vi "cRIO Vendor and Components Library.vi"() -> (0 "List of Modules":T4[](array[typedef])=[{"Module ID"=0, "Module Name"=""}, {"Module ID"=28836, "Module Name"="NI 9201"}, {"Module ID"=29089, "Module Name"="NI 9201 DSUB"}, {"Module ID"=29851, "Module Name"="NI 9201E"}, {"Module ID"=29853, "Module Name"="NI 9201E DSUB"}, {"Module ID"=28969, "Module Name"="NI 9203"}, {"Module ID"=29707, "Module Name"="NI 9203E"}, {"Module ID"=29162, "Module Name"="NI 9205"}, {"Module ID"=28970, "Module Name"="NI 9205 DSUB"}, {"Module ID"=29771, "Module Name"="NI 9205E"}, {"Module ID"=29163, "Module Name"="NI 9206"}, {"Module ID"=28835, "Module Name"="NI 9211"}, {"Module ID"=29706, "Module Name"="NI 9211E"}, {"Module ID"=29769, "Module Name"="NI 9213"}, {"Module ID"=29754, "Module Name"="NI 9213E"}, {"Module ID"=29934, "Module Name"="NI 9214"}, {"Module ID"=28838, "Module Name"="NI 9215"}, {"Module ID"=28981, "Module Name"="NI 9215 BNC"}, {"Module ID"=29709, "Module Name"="NI 9215E"}, {"Module ID"=29789, "Module Name"="NI 9215E BNC"}, {"Module ID"=28971, "Module Name"="NI 9217"}, {"Module ID"=29452, "Module Name"="NI 9219"}, {"Module ID"=29551, "Module Name"="NI 9219 LEMO"}, {"Module ID"=29761, "Module Name"="NI 9219E"}, {"Module ID"=29664, "Module Name"="NI 9220"}, {"Module ID"=30229, "Module Name"="NI 9220 DSUB"}, {"Module ID"=29841, "Module Name"="NI 9220E"}, {"Module ID"=28837, "Module Name"="NI 9221"}, {"Module ID"=29090, "Module Name"="NI 9221 DSUB"}, {"Module ID"=29852, "Module Name"="NI 9221E"}, {"Module ID"=29854, "Module Name"="NI 9221E DSUB"}, {"Module ID"=29571, "Module Name"="NI 9225"}, {"Module ID"=29704, "Module Name"="NI 9225E"}, {"Module ID"=29718, "Module Name"="NI 9227"}, {"Module ID"=29772, "Module Name"="NI 9227E"}, {"Module ID"=29437, "Module Name"="NI 9229"}, {"Module ID"=29544, "Module Name"="NI 9229 BNC"}, {"Module ID"=29725, "Module Name"="NI 9229E"}, {"Module ID"=28840, "Module Name"="NI 9233"}, {"Module ID"=29365, "Module Name"="NI 9234"}, {"Module ID"=29882, "Module Name"="NI 9234"}, {"Module ID"=30042, "Module Name"="NI 9234E"}, {"Module ID"=29482, "Module Name"="NI 9235"}, {"Module ID"=29898, "Module Name"="NI 9235E"}, {"Module ID"=29483, "Module Name"="NI 9236"}, {"Module ID"=29899, "Module Name"="NI 9236E"}, {"Module ID"=29123, "Module Name"="NI 9237"}, {"Module ID"=29604, "Module Name"="NI 9237 DSUB"}, {"Module ID"=29727, "Module Name"="NI 9237E"}, {"Module ID"=29774, "Module Name"="NI 9237E DSUB"}, {"Module ID"=29122, "Module Name"="NI 9239"}, {"Module ID"=29543, "Module Name"="NI 9239 BNC"}, {"Module ID"=29724, "Module Name"="NI 9239E"}, {"Module ID"=28839, "Module Name"="NI 9263"}, {"Module ID"=29545, "Module Name"="NI 9263 BNC"}, {"Module ID"=29726, "Module Name"="NI 9263E"}, {"Module ID"=29430, "Module Name"="NI 9264"}, {"Module ID"=29788, "Module Name"="NI 9264 DSUB"}, {"Module ID"=29767, "Module Name"="NI 9264E"}, {"Module ID"=29787, "Module Name"="NI 9264E DSUB"}, {"Module ID"=28972, "Module Name"="NI 9265"}, {"Module ID"=29762, "Module Name"="NI 9265E"}, {"Module ID"=29444, "Module Name"="NI 9375"}, {"Module ID"=29818, "Module Name"="NI 9375 DSUB"}, {"Module ID"=29802, "Module Name"="NI 9375E"}, {"Module ID"=29819, "Module Name"="NI 9375E DSUB"}, {"Module ID"=30274, "Module Name"="NI 9381"}, {"Module ID"=30272, "Module Name"="NI 9381 DSUB"}, {"Module ID"=28976, "Module Name"="NI 9401"}, {"Module ID"=29480, "Module Name"="NI 9402"}, {"Module ID"=28977, "Module Name"="NI 9403"}, {"Module ID"=29708, "Module Name"="NI 9403E"}, {"Module ID"=28829, "Module Name"="NI 9411"}, {"Module ID"=28831, "Module Name"="NI 9421"}, {"Module ID"=28974, "Module Name"="NI 9421 DSUB"}, {"Module ID"=29130, "Module Name"="NI 9422"}, {"Module ID"=28830, "Module Name"="NI 9423"}, {"Module ID"=28975, "Module Name"="NI 9425"}, {"Module ID"=29546, "Module Name"="NI 9426"}, {"Module ID"=30017, "Module Name"="NI 9426E"}, {"Module ID"=28828, "Module Name"="NI 9435"}, {"Module ID"=30128, "Module Name"="NI 9467"}, {"Module ID"=29907, "Module Name"="NI 9469"}, {"Module ID"=28833, "Module Name"="NI 9472"}, {"Module ID"=28978, "Module Name"="NI 9472 DSUB"}, {"Module ID"=28832, "Module Name"="NI 9474"}, {"Module ID"=29559, "Module Name"="NI 9475"}, {"Module ID"=28979, "Module Name"="NI 9476"}, {"Module ID"=29131, "Module Name"="NI 9477"}, {"Module ID"=29466, "Module Name"="NI 9478"}, {"Module ID"=29755, "Module Name"="NI 9478E"}, {"Module ID"=28834, "Module Name"="NI 9481"}, {"Module ID"=29705, "Module Name"="NI 9481E"}, {"Module ID"=29174, "Module Name"="NI 9485"}, {"Module ID"=29165, "Module Name"="NI 9505"}, {"Module ID"=29857, "Module Name"="NI 9505E"}, {"Module ID"=29645, "Module Name"="NI 9512"}, {"Module ID"=29646, "Module Name"="NI 9514"}, {"Module ID"=29648, "Module Name"="NI 9516"}, {"Module ID"=28980, "Module Name"="NI 9802"}, {"Module ID"=29171, "Module Name"="NI 9852"}, {"Module ID"=29007, "Module Name"="NI 9853"}, {"Module ID"=29820, "Module Name"="NI 9861"}, {"Module ID"=29821, "Module Name"="NI 9862"}, {"Module ID"=29824, "Module Name"="NI 9866"}, {"Module ID"=29445, "Module Name"="NI 9870"}, {"Module ID"=29759, "Module Name"="NI 9870E"}, {"Module ID"=29446, "Module Name"="NI 9871"}, {"Module ID"=29760, "Module Name"="NI 9871E"}, {"Module ID"=29826, "Module Name"="NI 9881"}, {"Module ID"=29827, "Module Name"="NI 9882"}, {"Module ID"=29850, "Module Name"="NI 9882"}, {"Module ID"=29765, "Module Name"="NI 9222"}, {"Module ID"=30515, "Module Name"="NI 9222 BNC"}, {"Module ID"=29766, "Module Name"="NI 9222E"}, {"Module ID"=29932, "Module Name"="NI 9223"}, {"Module ID"=30516, "Module Name"="NI 9223 BNC"}, {"Module ID"=29933, "Module Name"="NI 9223E"}, {"Module ID"=29729, "Module Name"="NI 9208"}, {"Module ID"=29868, "Module Name"="NI 9208 DSUB"}, {"Module ID"=29764, "Module Name"="NI 9208E"}, {"Module ID"=29867, "Module Name"="NI 9208E DSUB"}, {"Module ID"=29730, "Module Name"="NI 9207"}, {"Module ID"=29869, "Module Name"="NI 9207 DSUB"}, {"Module ID"=29866, "Module Name"="NI 9207E DSUB"}, {"Module ID"=29934, "Module Name"="NI 9214"}, {"Module ID"=30015, "Module Name"="NI 9232"}, {"Module ID"=30016, "Module Name"="NI 9232E"}, {"Module ID"=29717, "Module Name"="NI 9269"}, {"Module ID"=29773, "Module Name"="NI 9269E"}, {"Module ID"=29981, "Module Name"="NI 9501"}, {"Module ID"=29988, "Module Name"="NI 9501E"}, {"Module ID"=29982, "Module Name"="NI 9502"}, {"Module ID"=29989, "Module Name"="NI 9502E"}, {"Module ID"=30155, "Module Name"="NI 9795"}] {"Module ID" format="%.0x"}, 1 "List of Backplanes":T3(array[cluster])=[{"Backplane ID"=30549, "Backplane Name"=enum."cRIO-9030"}, {"Backplane ID"=30539, "Backplane Name"=enum."cRIO-9031"}, {"Backplane ID"=30517, "Backplane Name"=enum."cRIO-9033"}, {"Backplane ID"=30541, "Backplane Name"=enum."cRIO-9034"}, {"Backplane ID"=30683, "Backplane Name"=enum."cRIO-9035"}, {"Backplane ID"=30684, "Backplane Name"=enum."cRIO-9036"}, {"Backplane ID"=30649, "Backplane Name"=enum."cRIO-9038"}, {"Backplane ID"=30685, "Backplane Name"=enum."cRIO-9039"}, {"Backplane ID"=30528, "Backplane Name"=enum."cRIO-9063"}, {"Backplane ID"=30529, "Backplane Name"=enum."cRIO-9064"}, {"Backplane ID"=30530, "Backplane Name"=enum."cRIO-9065"}, {"Backplane ID"=30531, "Backplane Name"=enum."cRIO-9066"}, {"Backplane ID"=30532, "Backplane Name"=enum."cRIO-9067"}, {"Backplane ID"=30456, "Backplane Name"=enum."cRIO-9068"}, {"Backplane ID"=29127, "Backplane Name"=enum."cRIO-9072"}, {"Backplane ID"=29677, "Backplane Name"=enum."cRIO-9073"}, {"Backplane ID"=29341, "Backplane Name"=enum."cRIO-9074"}, {"Backplane ID"=30067, "Backplane Name"=enum."cRIO-9075"}, {"Backplane ID"=29991, "Backplane Name"=enum."cRIO-9076"}, {"Backplane ID"=29979, "Backplane Name"=enum."cRIO-9081"}, {"Backplane ID"=29980, "Backplane Name"=enum."cRIO-9082"}, {"Backplane ID"=28918, "Backplane Name"=enum."cRIO-9101"}, {"Backplane ID"=28766, "Backplane Name"=enum."cRIO-9102"}, {"Backplane ID"=28919, "Backplane Name"=enum."cRIO-9103"}, {"Backplane ID"=28920, "Backplane Name"=enum."cRIO-9104"}, {"Backplane ID"=29686, "Backplane Name"=enum."cRIO-9111"}, {"Backplane ID"=29687, "Backplane Name"=enum."cRIO-9112"}, {"Backplane ID"=29688, "Backplane Name"=enum."cRIO-9113"}, {"Backplane ID"=29689, "Backplane Name"=enum."cRIO-9114"}, {"Backplane ID"=29690, "Backplane Name"=enum."cRIO-9116"}, {"Backplane ID"=29691, "Backplane Name"=enum."cRIO-9118"}, {"Backplane ID"=30152, "Backplane Name"=enum."NI 9146"}, {"Backplane ID"=30540, "Backplane Name"=enum."NI 9147"}, {"Backplane ID"=29928, "Backplane Name"=enum."NI 9148"}, {"Backplane ID"=30542, "Backplane Name"=enum."NI 9149"}, {"Backplane ID"=30246, "Backplane Name"=enum."NI 9154"}, {"Backplane ID"=30247, "Backplane Name"=enum."NI 9155"}, {"Backplane ID"=30009, "Backplane Name"=enum."NI 9157"}, {"Backplane ID"=30010, "Backplane Name"=enum."NI 9159"}, {"Backplane ID"=29555, "Backplane Name"=enum."sbRIO-9601"}, {"Backplane ID"=29557, "Backplane Name"=enum."sbRIO-9602"}, {"Backplane ID"=30091, "Backplane Name"=enum."sbRIO-9605"}, {"Backplane ID"=30093, "Backplane Name"=enum."sbRIO-9606"}, {"Backplane ID"=29591, "Backplane Name"=enum."sbRIO-9611"}, {"Backplane ID"=29592, "Backplane Name"=enum."sbRIO-9612"}, {"Backplane ID"=30398, "Backplane Name"=enum."sbRIO-9623"}, {"Backplane ID"=30143, "Backplane Name"=enum."sbRIO-9626"}, {"Backplane ID"=29593, "Backplane Name"=enum."sbRIO-9631"}, {"Backplane ID"=29594, "Backplane Name"=enum."sbRIO-9632"}, {"Backplane ID"=30149, "Backplane Name"=enum."sbRIO-9633"}, {"Backplane ID"=30146, "Backplane Name"=enum."sbRIO-9636"}, {"Backplane ID"=29560, "Backplane Name"=enum."sbRIO-9641"}, {"Backplane ID"=29595, "Backplane Name"=enum."sbRIO-9642"}] {"Backplane ID" format="%.0x"}, 2 "List of Controllers":T1(array[cluster])=[{"Controller ID"=28767, "Controller Name"="cRIO-9002/9004"}, {"Controller ID"=29071, "Controller Name"="cRIO-9012"}, {"Controller ID"=29465, "Controller Name"="cRIO-9014"}, {"Controller ID"=29650, "Controller Name"="cRIO-9022/3"}, {"Controller ID"=29785, "Controller Name"="cRIO-9024/5"}, {"Controller ID"=30549, "Controller Name"="cRIO-9030"}, {"Controller ID"=30539, "Controller Name"="cRIO-9031"}, {"Controller ID"=30517, "Controller Name"="cRIO-9033"}, {"Controller ID"=30541, "Controller Name"="cRIO-9034"}, {"Controller ID"=30683, "Controller Name"="cRIO-9035"}, {"Controller ID"=30684, "Controller Name"="cRIO-9036"}, {"Controller ID"=30649, "Controller Name"="cRIO-9038"}, {"Controller ID"=30685, "Controller Name"="cRIO-9039"}, {"Controller ID"=30528, "Controller Name"="cRIO-9063"}, {"Controller ID"=30529, "Controller Name"="cRIO-9064"}, {"Controller ID"=30530, "Controller Name"="cRIO-9065"}, {"Controller ID"=30531, "Controller Name"="cRIO-9066"}, {"Controller ID"=30532, "Controller Name"="cRIO-9067"}, {"Controller ID"=30422, "Controller Name"="cRIO-9068"}, {"Controller ID"=29127, "Controller Name"="cRIO-9072"}, {"Controller ID"=29677, "Controller Name"="cRIO-9073"}, {"Controller ID"=29341, "Controller Name"="cRIO-9074"}, {"Controller ID"=29991, "Controller Name"="cRIO-9075/6"}, {"Controller ID"=30013, "Controller Name"="cRIO-9081/2"}, {"Controller ID"=29555, "Controller Name"="sbRIO-9601"}, {"Controller ID"=29557, "Controller Name"="sbRIO-9602"}, {"Controller ID"=30091, "Controller Name"="sbRIO-9605/6"}, {"Controller ID"=29591, "Controller Name"="sbRIO-9611"}, {"Controller ID"=29592, "Controller Name"="sbRIO-9612"}, {"Controller ID"=30142, "Controller Name"="sbRIO-9623"}, {"Controller ID"=30145, "Controller Name"="sbRIO-9626"}, {"Controller ID"=29593, "Controller Name"="sbRIO-9631"}, {"Controller ID"=29594, "Controller Name"="sbRIO-9632"}, {"Controller ID"=30149, "Controller Name"="sbRIO-9633"}, {"Controller ID"=30146, "Controller Name"="sbRIO-9636"}, {"Controller ID"=29560, "Controller Name"="sbRIO-9641"}, {"Controller ID"=29595, "Controller Name"="sbRIO-9642"}] {"Controller ID" format="%.0x"}, 3 "List of Vendors":cluster{"Vendor ID":u16, "Vendor Name":string}[](array[cluster])=[{"Vendor ID"=0, "Vendor Name"=""}, {"Vendor ID"=4243, "Vendor Name"="National Instruments"}, {"Vendor ID"=44884, "Vendor Name"="AFT Atlas Fahrzeugtechnik"}, {"Vendor ID"=18193, "Vendor Name"="S.E.A. Datentechnik"}, {"Vendor ID"=56852, "Vendor Name"="Drivven"}, {"Vendor ID"=21226, "Vendor Name"="Bluetechnix"}, {"Vendor ID"=59499, "Vendor Name"="SET"}, {"Vendor ID"=8211, "Vendor Name"="COMSOFT"}, {"Vendor ID"=12507, "Vendor Name"="Averna"}] {"Vendor ID" format="%.0x"})   [LabVIEW 2016]
uses:
  Module/Controls/ModuleInformation.ctl
  Module/Module.lvclass
  Chassis/Controls/ChassisInformation.ctl
  Chassis/Chassis.lvclass
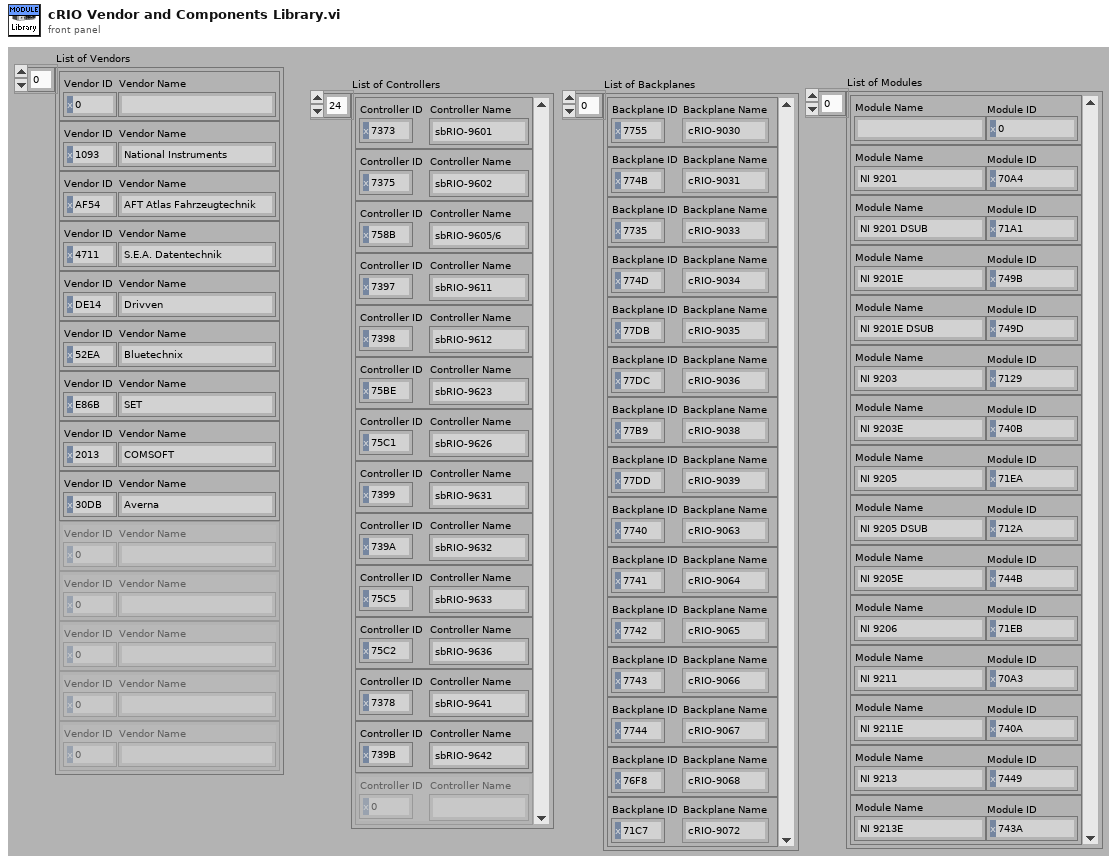
[diagram p1: front panel]
types:
  T1 = cluster{"Controller ID":u16, "Controller Name":string}[]
  T2 = typedef "cRIO Backplanes.ctl" = enum16{"<Undefined>", "cRIO-9030", "cRIO-9031", "cRIO-9033", "cRIO-9034", "cRIO-9035", "cRIO-9036", "cRIO-9038", "cRIO-9039", "cRIO-9063", "cRIO-9064", "cRIO-9065", "cRIO-9066", "cRIO-9067", "cRIO-9068", "cRIO-9072", "cRIO-9073", "cRIO-9074", "cRIO-9075", "cRIO-9076", "cRIO-9081", "cRIO-9082", "cRIO-9101", "cRIO-9102", "cRIO-9103", "cRIO-9104", "cRIO-9111", "cRIO-9112", "cRIO-9113", "cRIO-9114", "cRIO-9116", "cRIO-9118", "NI 9146", "NI 9147", "NI 9148", "NI 9149", "NI 9154", "NI 9155", "NI 9157", "NI 9159", "myRIO-1900", "myRIO-1950", "sbRIO-9601", "sbRIO-9602", "sbRIO-9605", "sbRIO-9606", "sbRIO-9611", "sbRIO-9612", "sbRIO-9623", "sbRIO-9626", "sbRIO-9631", "sbRIO-9632", "sbRIO-9633", "sbRIO-9636", "sbRIO-9641", "sbRIO-9642"}
  T3 = cluster{"Backplane ID":u16, "Backplane Name":T2}[]
  T4 = typedef "cRIO Module Code.ctl" = cluster{"Module ID":u16, "Module Name":string}
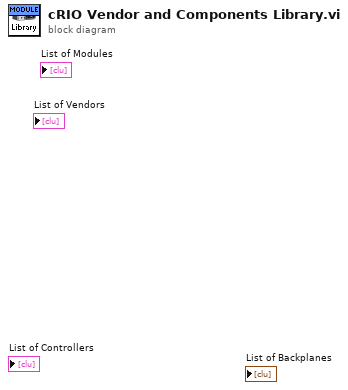
[diagram p0: block diagram]
diagram:
